vi "SP Determine Channel Type From Name.vi"(10 "Channel Name":string) -> (2 "Channel Type":T1=enum."Data")   [LabVIEW 2011]
uses:
  TypeDefs/SP Channel Type.ctl
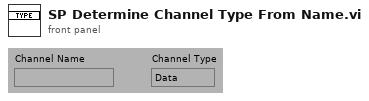
[diagram p1: front panel]
types:
  T1 = typedef "SP Channel Type.ctl" = enum16{"Frequency", "Data", "Limit", "Adapter", "Memory", "Value", "Value Limit"}
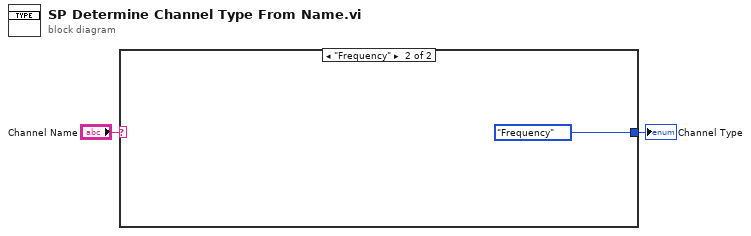
[diagram p0: block diagram]
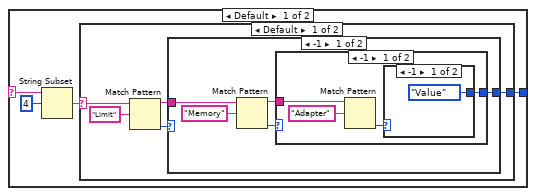
[diagram p2: hidden frame]
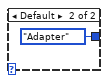
[diagram p3: hidden frame]
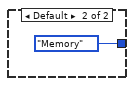
[diagram p4: hidden frame]
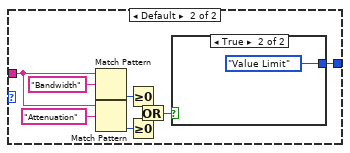
[diagram p5: hidden frame]
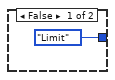
[diagram p6: hidden frame]
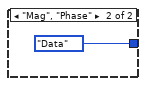
[diagram p7: hidden frame]
diagram:
  n1 = case shown="\"Frequency\"" "Channel Name" {
    selector: "Channel Name" -> [w5 _]
    tunnel: [w3 SP_Channel_Type."Frequency" ("Channel Type")] -> w1
    frame Default {
      n2 = String Subset(string=w5, offset (0)=4) -> (substring=w4:string)  [unwired: 1 out]
      n3 = case shown="Default" w4 {
        selector: w4 -> [w10 _]
        tunnel: [w7 SP_Channel_Type."Data" ("Channel Type")] -> w3
        frame Default {
          n4 = Match Pattern(string=w10, regular expression="Limit") -> (before substring=w8:string, offset past match=w9:i32)  [unwired: 3 out]
          n5 = case shown="-1" w9 {
            tunnel: w8 -> [w15 w30]
            tunnel: [w12 w24] -> w7
            frame -1 {
              n6 = Match Pattern(string=w15, regular expression="Memory") -> (before substring=w13:string, offset past match=w14:i32)  [unwired: 3 out]
              n7 = case shown="-1" w14 {
                tunnel: w13 -> [w19 _]
                tunnel: [w17 SP_Channel_Type."Memory" ("Channel Type")] -> w12
                frame -1 {
                  n8 = Match Pattern(string=w19, regular expression="Adapter") -> (offset past match=w18:i32)  [unwired: 4 out]
                  n9 = case shown="-1" w18 {
                    tunnel: [SP_Channel_Type."Value" ("Channel Type") SP_Channel_Type."Adapter" ("Channel Type")] -> w17
                    frame -1 {
                    }
                    frame Default {
                    }
                  }
                }
                frame Default {
                }
              }
            }
            frame Default {
              n10 = Match Pattern(string=w30, regular expression="Bandwidth") -> (offset past match=w29:i32)  [unwired: 4 out]
              n11 = Match Pattern(string=w30, regular expression="Attenuation") -> (offset past match=w28:i32)  [unwired: 4 out]
              n12 = Greater Or Equal To 0?(x=w29) -> (x >= 0?=w27:bool)
              n13 = Greater Or Equal To 0?(x=w28) -> (x >= 0?=w26:bool)
              n14 = Or(x=w27, y=w26) -> (x .or. y?=w25:bool)
              n15 = case shown="True" w25 {
                tunnel: [SP_Channel_Type."Limit" ("Channel Type") SP_Channel_Type."Value Limit" ("Channel Type")] -> w24
                frame False {
                }
                frame True {
                }
              }
            }
          }
        }
        frame "Mag", "Phase" {
        }
      }
    }
    frame "Frequency" {
    }
  }
  "Channel Type" <- w1
